vi "Transceiver Interface.New.vi"(5 "FIFO Debug Flags":refnum<class "FIFO Flags.lvclass">, 7 "fifo depths (10)":u32=10, 8 "error in (no error)":errorcluster, 10 "error size (512 B)":T1=enum."512-byte", 11 "Transceiver Interface type":refnum<class "Transceiver Interface.lvclass">) -> (0 "error out":errorcluster, 3 "Transceiver Interface":refnum<class "Transceiver Interface.lvclass">)   [LabVIEW 2017, in "DSF Core.lvlib" / "Transceiver Interface.lvclass"]
uses:
  Transceiver Interface.lvclass
  C:/Git/DSF/dsf core/Source/Engine/Classes/Interface/Interface.lvclass
  Interface.Error Queue.Sizes.ctl
  Debug/FIFO Flags.lvclass
  Interface.lvclass
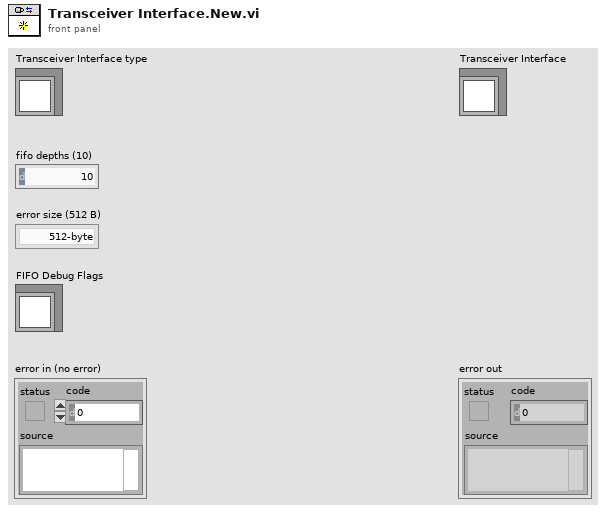
[diagram p1: front panel]
types:
  T1 = typedef "DSF Core.lvlib/Interface.lvclass/Interface.Error Queue.Sizes.ctl" = enum16{"256-byte", "512-byte", "1024-byte"}
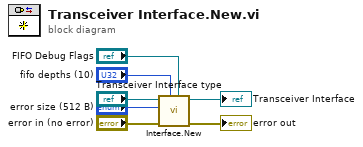
[diagram p0: block diagram]
diagram:
  n1 = call "Interface.New.vi"("FIFO Debug Flags"="FIFO Debug Flags", "fifo/queue depths (10)"="fifo depths (10)", "error in (no error)"="error in (no error)", "error size (512 B)"="error size (512 B)", "Interface type"="Transceiver Interface type") -> ("error out"=→"error out":errorcluster, "Interface"=→"Transceiver Interface":refnum<class "Transceiver Interface.lvclass">)  [unwired: 5 in]
